vi "Write List of Test Names.vi"(2 "Results":T1[](array[typedef]), 5 "error in (no error)":errorcluster, 6 "file path (use dialog)":path=path "C:/SSP/Snap-On_GEP/trunk/Software/Log Results/TEST NAMES LOG.csv") -> (19 "error out":errorcluster)   [LabVIEW 2015]
uses:
  Test Result.ctl
panel:
  out "concatenated string":string
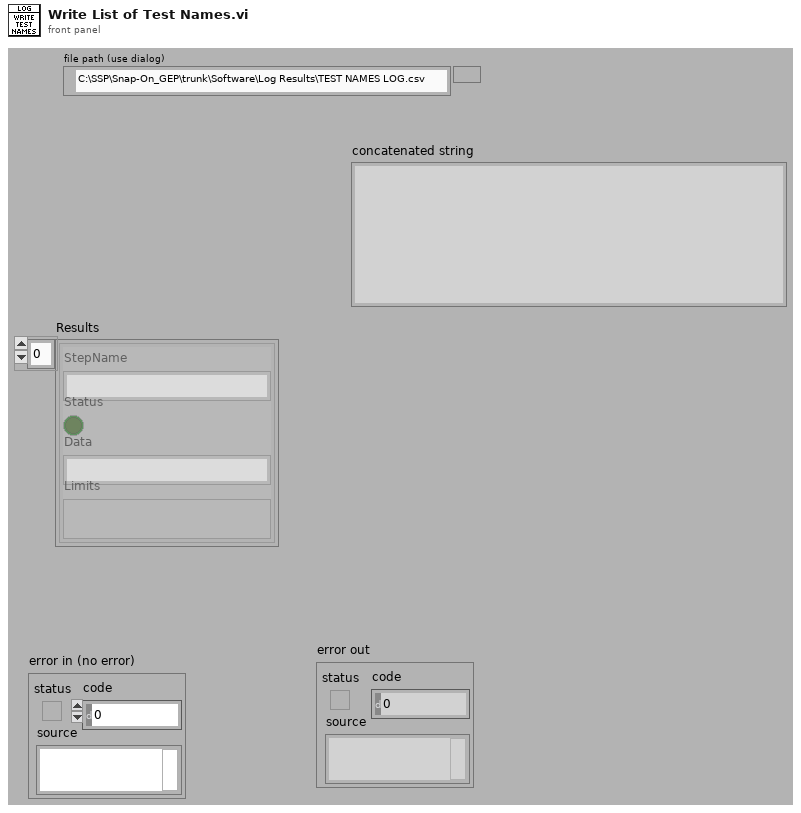
[diagram p1: front panel]
types:
  T1 = typedef "Test Result.ctl" = cluster{"StepName":string, "Status":bool, "Data":string, "Limits":variant}
  T2 = enum16{"open", "replace", "create", "open or create", "replace or create", "replace or create with confirmation"}
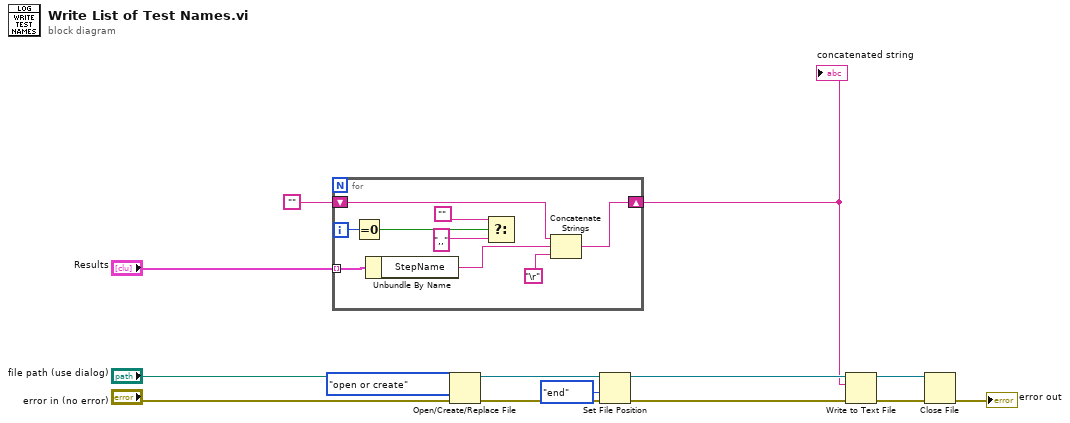
[diagram p0: block diagram]
diagram:
  n1 = for {
    tunnel: "Results" -> [w23] mode=indexing
    shift-right: [w21] -> w2
    shift-left: "" -> [w19]
    i -> [w18]
    n2 = Equal To 0?(x=w18) -> (x = 0?=w17:bool)
    n3 = Unbundle By Name(w23) -> ("StepName"=w22:string)
    n4 = Select(t="", s=w17, f=",," ("string")) -> ()  [unwired: 1 out]
    n5 = Concatenate Strings(w19, w22, "\r") -> (w21:string)
  }
  "concatenated string" <- w2
  n6 = Open/Create/Replace File(file path (use dialog)="file path (use dialog)", error in="error in (no error)", operation (0:open)=T2."open or create") -> (refnum out=w11:refnum<file>, error out=w9:errorcluster)  [unwired: 3 in, 1 out]
  n7 = Set File Position(refnum=w11, from (0:start)=enum16{"start", "end", "current"}."end", error in=w9) -> (refnum out=w10:refnum<file>, error out=w8:errorcluster)  [unwired: 1 in]
  n8 = Write to Text File(file (use dialog)=w10, text=w2, error in=w8) -> (refnum out=w3:refnum<file>, error out=w5:errorcluster)  [unwired: 1 in, 1 out]
  n9 = Close File(refnum=w3, error in=w5) -> (error out=→"error out":errorcluster)  [unwired: 1 out]
